vi "_emi_GFV stop a loop so it can reset.vi"(0 "Loop Index/Numb":u16, 1 "Action(Get Index)":T1=enum."Get index", 7 "Value In":bool, 11 "error in (no error)":errorcluster) -> (4 "Index out":u16, 8 "Value Out":bool, 10 "Size":i32, 15 "error out":errorcluster)   [LabVIEW 2011]
uses:
  _emi_Loop control int action.ctl
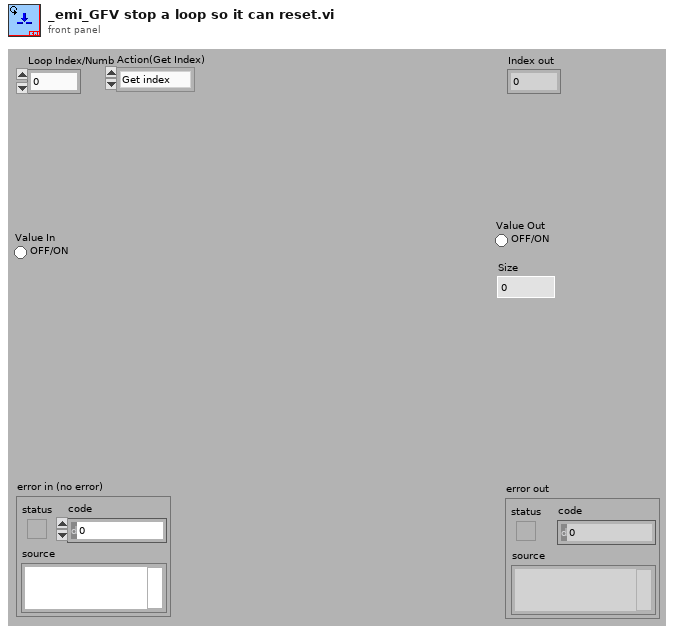
[diagram p1: front panel]
types:
  T1 = typedef "_emi_Loop control int action.ctl" = enum16{"Init index", "Get index", "Set index", "Get Size"}
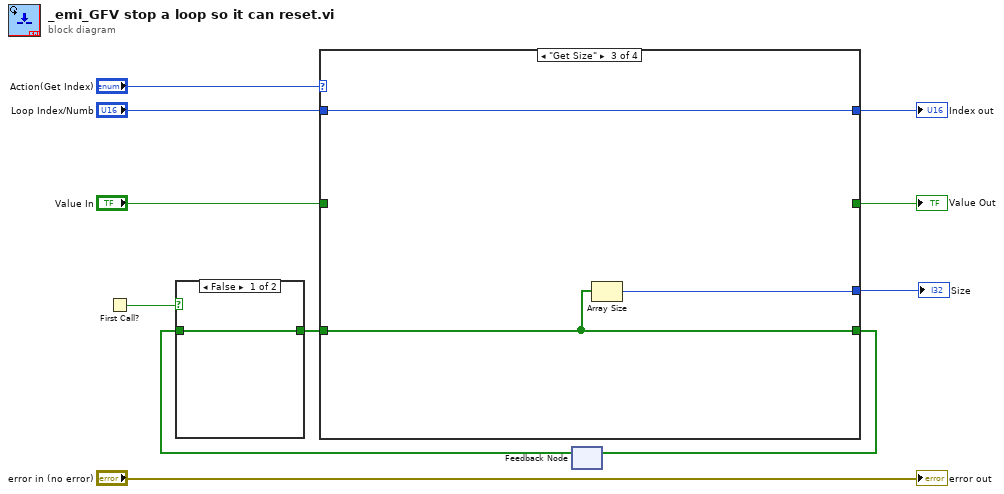
[diagram p0: block diagram]
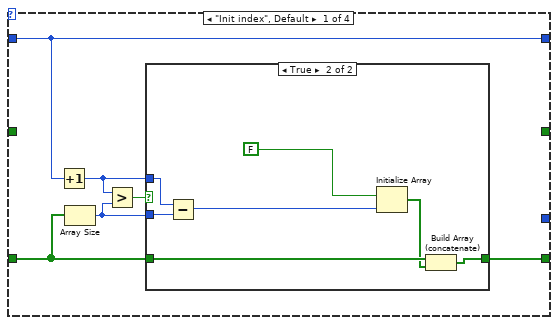
[diagram p2: hidden frame]
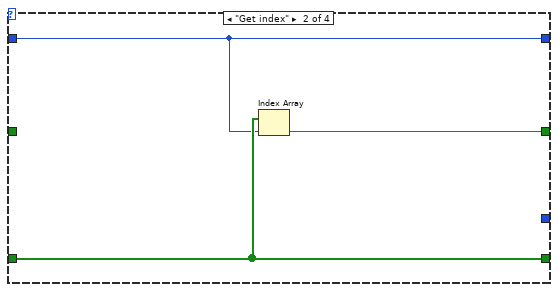
[diagram p4: hidden frame]
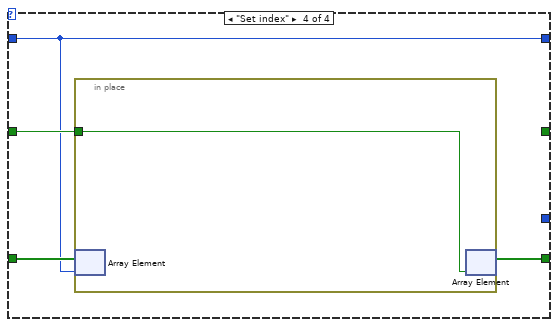
[diagram p5: hidden frame]
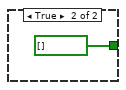
[diagram p6: hidden frame]
diagram:
  n1 = First Call?() -> (First Call?: T/F=w11:bool)
  n2 = feedback #1() -> (w5:bool[])  [unwired: 1 in]
  n3 = case shown="False" w11 {
    tunnel: [w12 bool[] []] -> w6
    tunnel: w5 -> [w12 _]
    frame False {
    }
    frame True {
    }
  }
  n4 = case shown="\"Get Size\"" "Action(Get Index)" {
    tunnel: [w19 w29 w33 w34] -> w10
    tunnel: "Loop Index/Numb" -> [w19 w29 w33 w34]
    tunnel: [w15 w30 w32 w36] -> w7
    tunnel: w6 -> [w14 w30 w32 w37]
    tunnel: [_ w28 _ _] -> w4
    tunnel: "Value In" -> [_ _ _ w35]
    tunnel: [_ _ w31 _] -> w1
    frame "Init index", Default {
      n5 = Increment(x=w19) -> (x+1=w16:u16)
      n6 = Array Size(array=w14) -> (size(s)=w17:i32)
      n7 = Greater?(x=w16, y=w17) -> (0:w18:bool)
      n8 = case shown="True" w18 {
        tunnel: w17 -> [_ w26]
        tunnel: w16 -> [_ w27]
        tunnel: [w20 w21] -> w15
        tunnel: w14 -> [w20 w23]
        frame False {
        }
        frame True {
          n9 = Subtract(x=w27, y=w26) -> (x-y=w25:i32)
          n10 = Initialize Array(FALSE, w25) -> (w22:bool[])
          n11 = Build Array (concatenate)(w23, w22) -> (w21:bool[])
        }
      }
    }
    frame "Get index" {
      n12 = Index Array(array=w30, index=w29) -> (element=w28:bool)
    }
    frame "Get Size" {
      n13 = Array Size(array=w32) -> (size(s)=w31:i32)
    }
    frame "Set index" {
      n14 = in-place {
        in-place-border: w35 -> [w38]
        n15 = in-place-array #2(w37, w34) -> ()  [unwired: 1 out]
        n16 = in-place-array #2(w38) -> (w36:bool[])  [unwired: 1 out]
      }
    }
  }
  "Index out" <- w10
  "Value Out" <- w4
  "Size" <- w1
  n17 = feedback-in #1(w7) -> ()
  "error out" <- "error in (no error)"
